vi "Convert Pressure (mbar) to Altitude (m).vi"(10 "Altimeter Setting (mbar)":dbl=1013.25, 11 "Pressure (mbar)":dbl) -> (3 "Altitude (m)":dbl)   [LabVIEW 2020, in "LPS Barometric Pressure Sensor.lvclass"]
doc: "Converts pressure in mbar to altitude in meters, using 1976 US Standard Atmosphere model (only applicable up to height of 11km/36,000ft). If altimeter setting (QNH, barometric pressure adjusted to sea level) is given, this function returns an indicated altitude compensated for actual regional pressure; otherwise, it returns the pressure altitude above the standard pressure level of 1013.25mbar or 29.9213 inHg."
uses:
  LPS Barometric Pressure Sensor.lvclass
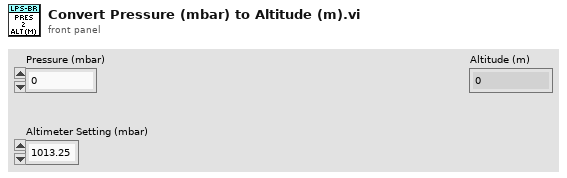
[diagram p1: front panel]
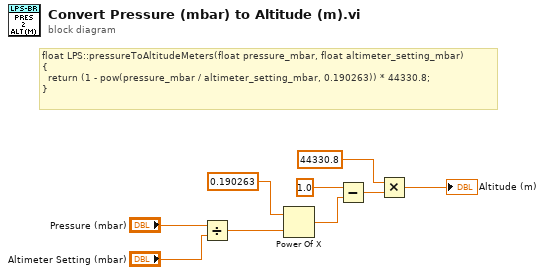
[diagram p0: block diagram]
diagram:
  # "float LPS::pressureToAltitudeMeters(float pressure_mbar, float altimeter_setting_mbar)\n{\n  return (1 - pow(pressure_mbar / altimeter_setting_mbar, 0.190263)) * 44330.8;\n}"
  n1 = Divide(x="Pressure (mbar)", y="Altimeter Setting (mbar)") -> (x/y=w6:dbl)
  n2 = Power Of X(1:w6, 2:0.190263 ("x")) -> (0:w4:dbl)
  n3 = Subtract(x=1.0, y=w4) -> (x-y=w3:dbl)
  n4 = Multiply(x=44330.8, y=w3) -> (x*y=→"Altitude (m)":dbl)
